vi "EE_InitializeDataAcquisition.vi"(0 "EmotivEpocHeadsetControls in":refnum<class "EmotivEpocHeadsetControls.lvclass">, 11 "error in (no error)":errorcluster) -> (4 "EmotivEpocHeadsetControls out":refnum<class "EmotivEpocHeadsetControls.lvclass">, 15 "error out":errorcluster)   [LabVIEW 2016, in "Emotiv Epoc.lvlib" / "EmotivEpocHeadsetControls.lvclass"]
uses:
  EmotivEpocHeadsetControls.lvclass
  EmotivEpocHeadsetControls.lvclass/EmotivEpocHeadsetControls.ctl
panel:
  # "This VI is a part of BCI Design library, http://www.ru-bci.org \nCopyright © 2020, Sotnikov Peter, All rights reserved. License: GNU GPLv3"
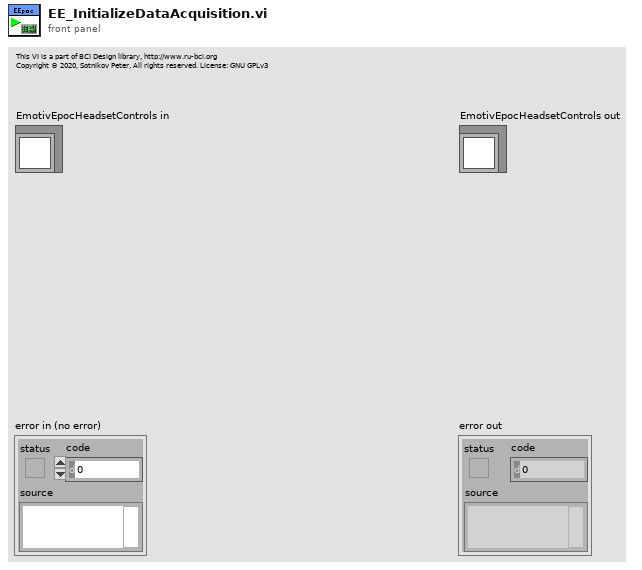
[diagram p1: front panel]
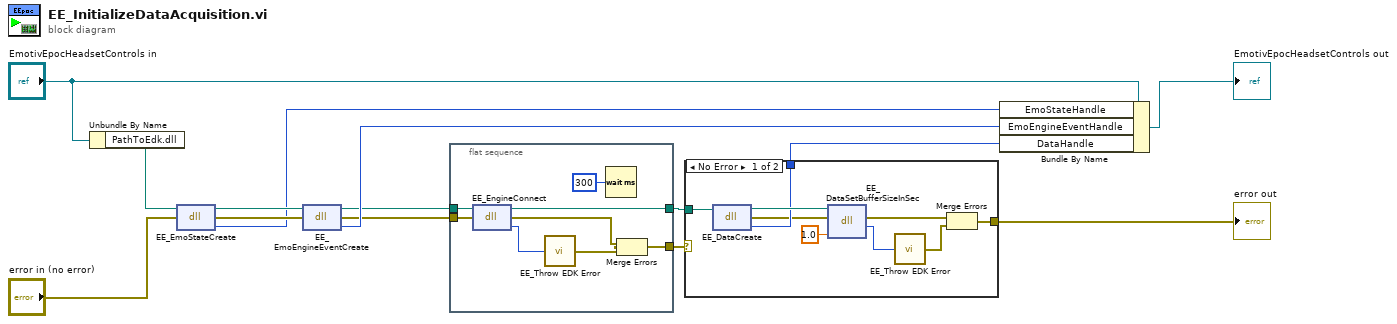
[diagram p0: block diagram]
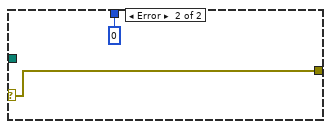
[diagram p2: hidden frame]
diagram:
  n1 = Unbundle By Name("EmotivEpocHeadsetControls in") -> ("PathToEdk.dll"=w1:path)
  n2 = dll-call lib="C:/Program Files/Emotiv Development Kit_v1.0.0.3-PREMIUM/edk.dll" fn="EE_EmoStateCreate"(path in=w1, error in="error in (no error)") -> (path out=w12:path, error out=w11:errorcluster, "EmoStateHandle"=w8:i64)  [unwired: 1 in]
  n3 = dll-call lib="?" fn="EE_EmoEngineEventCreate"(path in=w12, error in=w11) -> (path out=w5:path, error out=w6:errorcluster, "EmoEngineEventHandle"=w7:i64)  [unwired: 1 in]
  n4 = flat-sequence {
    tunnel: w6 -> [w21]
    tunnel: w5 -> [w20]
    tunnel: [w19] -> w4
    tunnel: [w18] -> w3
    frame #0 {
      n5 = dll-call lib="?" fn="EE_EngineConnect"(path in=w20, error in=w21) -> (path out=w19:path, error out=w16:errorcluster, "EDK_ERROR_CODE"=w17:i32)  [unwired: 1 in]
      n6 = call "EE_Throw EDK Error.vi"("edkErrorCode"=w17) -> ("edkErroCode"=w22:errorcluster)
      n7 = Wait (ms)(milliseconds to wait=u32 300) -> ()  [unwired: 1 out]
      n8 = Merge Errors(w16, w22) -> (w18:errorcluster)
    }
  }
  n9 = case shown="No Error" w3 {
    selector: w3 -> [_ w32]
    tunnel: [w29 i64 0 ("DataHandle")] -> w14
    tunnel: w4 -> [w27 _]
    tunnel: [w25 w32] -> w2
    frame No Error {
      n10 = dll-call lib="?" fn="EE_DataCreate"(path in=w27) -> (path out=w30:path, error out=w28:errorcluster, "DataHandle"=w29:i64)  [unwired: 2 in]
      n11 = dll-call lib="?" fn="EE_DataSetBufferSizeInSec"(path in=w30, error in=w28, "bufferSizeInSec"=sgl 1.0) -> (error out=w23:errorcluster, "EDK_ERROR_CODE"=w26:i32)  [unwired: 2 in, 1 out]
      n12 = call "EE_Throw EDK Error.vi"("edkErrorCode"=w26) -> ("edkErroCode"=w24:errorcluster)
      n13 = Merge Errors(w23, w24) -> (w25:errorcluster)
    }
    frame Error {
    }
  }
  "error out" <- w2
  n14 = Bundle By Name(cluster="EmotivEpocHeadsetControls in", "EmoStateHandle"=w8, "EmoEngineEventHandle"=w7, "DataHandle"=w14) -> (→"EmotivEpocHeadsetControls out":refnum<class "EmotivEpocHeadsetControls.lvclass">)
